vi "Make Nx512 Array.vi"(1 "1D Flat Array":bool[](array[boolean])) -> (0 "2D Nx512 Array":bool[][](array[boolean]))   [LabVIEW 2014]
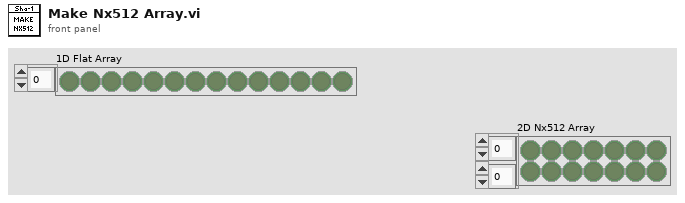
[diagram p1: front panel]
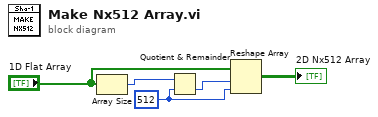
[diagram p0: block diagram]
diagram:
  w1 = 512 ("y")
  n1 = Array Size(array="1D Flat Array") -> (size(s)=w5:i32)
  n2 = Quotient & Remainder(x=w5, y=w1) -> (floor(x/y)=w2:i32)  [unwired: 1 out]
  n3 = Reshape Array("1D Flat Array", w2, w1) -> (→"2D Nx512 Array":bool[][])
